vi "MU Get Version Patch.vi"(8 "error in (no error)":errorcluster) -> (0 "error out (no error)":errorcluster, 3 "versionPatch":u16)   [LabVIEW 2017, in "MU_3SL_interface.lvlib"]
uses:
  MU_3SL_interface.lvlib
  lib/MU_3SL_interface.dll
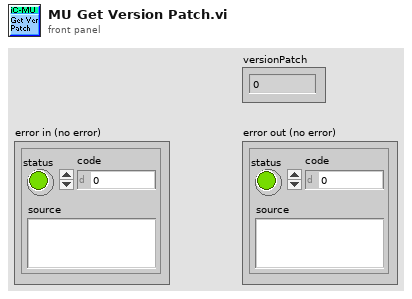
[diagram p1: front panel]
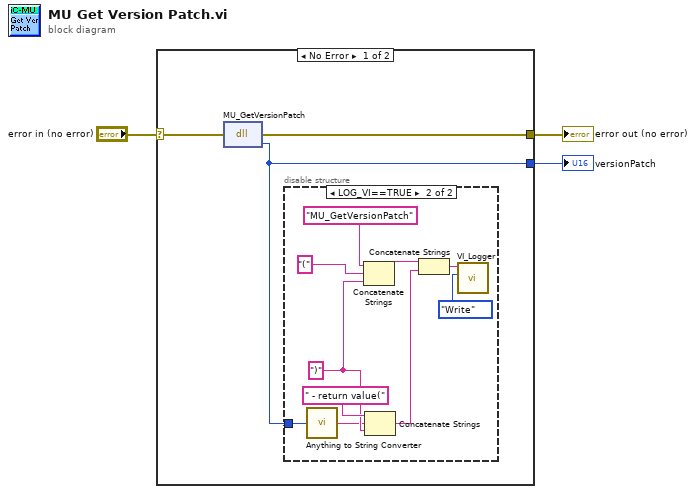
[diagram p0: block diagram]
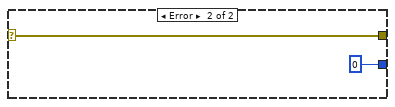
[diagram p3: hidden frame]
diagram:
  n1 = case shown="No Error" "error in (no error)" {
    selector: "error in (no error)" -> [w6 w18]
    tunnel: [w5 w18] -> w3
    tunnel: [w4 u16 0 ("versionMajor")] -> w1
    frame No Error {
      n2 = dll-call lib="C:/Users/bes/AppData/Roaming/work/mu_9so/icsubmodules/soft_mu_3sl_master/lv_interface/lib/MU_3SL_interface**.*" fn="MU_GetVersionPatch"(error in=w6) -> (error out=w5:errorcluster, "versionPatch"=w4:u16)  [unwired: 2 in, 1 out]
      n3 = disable-structure shown="LOG_VI==TRUE" {
        disable-tunnel: w4 -> [_ w8]
        frame condition #0 {
        }
        frame condition #1 (active) {
          w9 = ")" ("string")
          n4 = call "Anything to String Converter.vi"("anything"=w8) -> ("String"=w7:string)
          n5 = Concatenate Strings("MU_GetVersionPatch" ("Info in"), "(" ("string"), w9) -> (w14:string)
          n6 = Concatenate Strings(" - return value(" ("string"), w7, w9) -> (w13:string)
          n7 = Concatenate Strings(w14, w13) -> (w12:string)
          n8 = call "VI_Logger.vi"("Action (Read)"=enum16{"Write", "Read"}."Write", "Info in"=w12) -> ()  [unwired: 8 in, 2 out]
        }
      }
    }
    frame Error {
    }
  }
  "error out (no error)" <- w3
  "versionPatch" <- w1
